vi "Main.vi"() -> ()   [LabVIEW 2021]
doc: "Use this template to build a simple state machine design pattern. Each state executes code and determines which state to transition to."
uses:
  controls/UI Data.ctl
  Serial - Settings.ctl
  controls/Sensor parameters.ctl
  controls/State.ctl
  dd997a8f-e2f9-4ff0-8e35-442db1fc508d.vi
  22f98573-57d9-4471-b3a5-586873744a38.vi
  <vilib>/Instr/_visa.llb/VISA Configure Serial Port (Instr).vi
  <vilib>/Utility/file.llb/Write Delimited Spreadsheet (string).vi
panel:
  in  "AUTOMATICKE NASTAVENI \nPARAMETRU":enum16{"OFF", "Presnost", "Rychlost"}(ring)
  in  "Tab Control":T1(tab)
  in  "Ukladani":u16(ring) items=[".csv", ".tdms"]
  in  "Celkovy pocet mereni":u32=20 step=10
  in  "Pocet mereni na prumer":u32=5 min=1 max=20
  in  "Pocet mereni za sekundu":dbl=4.0 min=1.0 max=5.0
  in  "Save measurement to:":path=path "TEST3"
  in  "VISA resource name 34450A":refnum<visa-resource-name>="key"
  in  "delay before read 34450A":u32=500
  in  "Rozsah 34450A":T2(ring)=enum."10 V"
  in  "Rozliseni 34450A":enum16{"4_1/2 fast", "4_1/2 slow", "5_1/2 fast"}(ring)
  in  "VISA resource name 34401A":refnum<visa-resource-name>="COM7"
  in  "delay before read 34401A":u32=500
  in  "Rozliseni 34401A":T3(ring)
  in  "Rozsah 34401A":enum16{"10 mA", "100 mA", "1 A", "3 A"}(ring)
  in  "Serial Settings 34401A":T4={"baud rate"=9600, "data bits"=8, "parity"=enum."None", "stop bits"=10, "flow control"=0} {"flow control" items=["None"=0, "XON/XOFF"=1, "RTS/CTS"=2, "DTR/DSR"=4]; "stop bits" items=["1.0"=10, "1.5"=15, "2.0"=20]; "data bits" min=5 max=8 step=1; "baud rate" items=["75"=75, "110"=110, "134"=134, "150"=150, "300"=300, "600"=600, "1200"=1200, "1800"=1800, "2400"=2400, "4800"=4800, "7200"=7200, "9600"=9600, "14400"=14400, "19200"=19200, "28800"=28800, "38400"=38400, "56000"=56000, "57600"=57600, "115200"=115200, "128000"=128000, "230400"=230400]}
  out "Odhad konce mereni":timestamp
  out "Start mereni":timestamp
  in  "Stop mereni":bool
  out "Probiha mereni":u8(slide) scale=0.0..1.0
  in  "Sensor parameters":T5
  in  "Start mereni":bool
  out "Prumerna teplota":waveform(dbl)(graph)={"t0"=timestamp(3860297685.555485 s since 1904-01-01), "dt"=1.2529971599578857, "Y"=[-inf, -inf, -inf, -inf, nan]}
  out "Table":string[][](table)=[["Casy prumeru", "4/29/2026 10:54:45 AM", "4/29/2026 10:54:46 AM", "4/29/2026 10:54:48 AM", "4/29/2026 10:54:49 AM", "2/28/1965 5:27:24 PM"], ["Prumery napeti [V]", "-0.000417", "-0.000469", "-0.000557", "-0.000539", "NaN"], ["Prumery proudu [A]", "-0.000000", "0.000000", "-0.000000", "-0.000001", "NaN"], ["Prumery odporu [Ohm]", "-10579.900593", "-10579.900593", "-10579.900593", "-10579.900593", "NaN"], ["Prumery teploty [°C]", "-Inf", "-Inf", "-Inf", "-Inf", "NaN"], ["Nejistoty teplot [°C]", "NaN", "NaN", "NaN", "NaN", "NaN"]]
  in  "stop":bool
  in  "Data":T6={"VISA resource name 34401A"="COM1", "Serial Settings 34401A"={"baud rate"=9600, "data bits"=8, "parity"=enum."None", "stop bits"=10, "flow control"=0}, "VISA resource name 34450"="COM1", "VISA OUT 34401A"="", "VISA OUT 34450"="", "Delay before read 34401A"=0, "Delay before read 34450"=0, "Pocet mereni za sekundu"=1.0, "Celkovy pocet mereni"=1, "Pocet mereni na prumer"=1, "Rozliseni 34401A"=enum."4_1/2 fast", "Rozliseni 34450"=enum."5_1/2 fast", "AUTOMATICKE NASTAVENI \nPARAMETRU"=enum."OFF", "Namerene napeti"=[], "Namerene proudy"=[], "Prumery napeti"=[], "Prumery proudu"=[], "Namerene odpory"=[], "Namerene teploty"=[], "Prumery odporu"=[], "Prumery teplot"=[], "Rozsah 34401A"=enum."10 mA", "Rozsah 34450"=enum."100 mV", "Sensor parameters"={"Sensor type"="", "Sensor constant"=0.0}, "Casy mereni"=[], "Casy prumerovani"=[], "Nejistoty teplot"=[]} {"Pocet mereni na prumer" min=1; "Celkovy pocet mereni" min=1 max=5; "Serial Settings 34401A"."flow control" items=["None"=0, "XON/XOFF"=1, "RTS/CTS"=2, "DTR/DSR"=4]; "Serial Settings 34401A"."stop bits" items=["1.0"=10, "1.5"=15, "2.0"=20]; "Serial Settings 34401A"."data bits" min=5 max=8 step=1; "Serial Settings 34401A"."baud rate" items=["75"=75, "110"=110, "134"=134, "150"=150, "300"=300, "600"=600, "1200"=1200, "1800"=1800, "2400"=2400, "4800"=4800, "7200"=7200, "9600"=9600, "14400"=14400, "19200"=19200, "28800"=28800, "38400"=38400, "56000"=56000, "57600"=57600, "115200"=115200, "128000"=128000, "230400"=230400]}
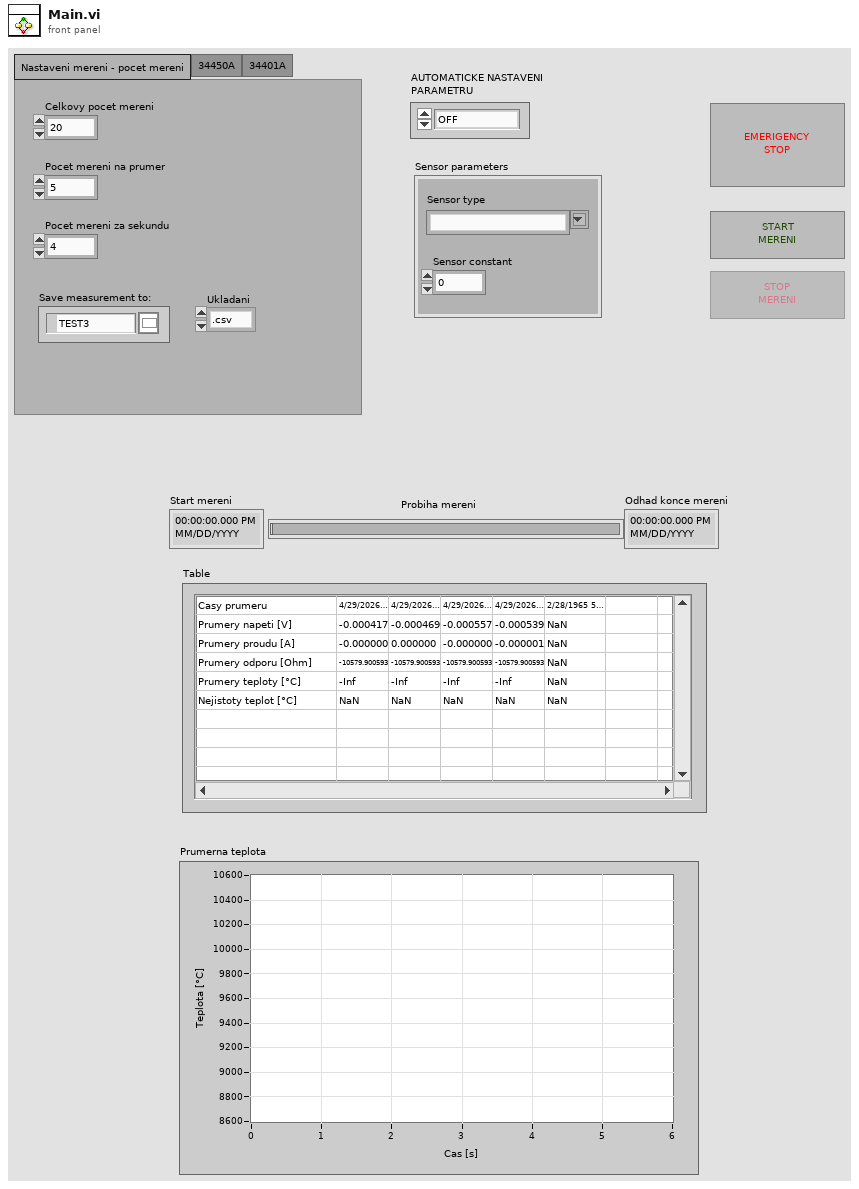
[diagram p1: front panel]
types:
  T1 = enum32{"Nastaveni mereni - pocet mereni", "34450A", "34401A"}
  T2 = enum16{"100 mV", "1 V", "10 V", "100 V", "1000 V"}
  T3 = enum16{"4_1/2 fast", "4_1/2 slow", "5_1/2 fast", "5_1/2 slow", "6_1/2 fast", "6_1/2 slow"}
  T4 = typedef "Serial - Settings.ctl" = cluster{"baud rate":u32, "data bits":u16, "parity":enum16{"None", "Odd", "Even", "Mark", "Space"}, "stop bits":u16, "flow control":u16}
  T5 = typedef "Sensor parameters.ctl" = cluster{"Sensor type":string, "Sensor constant":dbl}
  T6 = typedef "UI Data.ctl" = cluster{"VISA resource name 34401A":refnum<visa-resource-name>, "Serial Settings 34401A":T4, "VISA resource name 34450":refnum<visa-resource-name>, "VISA OUT 34401A":refnum<visa-resource-name>, "VISA OUT 34450":refnum<visa-resource-name>, "Delay before read 34401A":u32, "Delay before read 34450":u32, "Pocet mereni za sekundu":dbl, "Celkovy pocet mereni":u32, "Pocet mereni na prumer":u32, "Rozliseni 34401A":enum16{"4_1/2 fast", "4_1/2 slow", "5_1/2 fast", "5_1/2 slow", "6_1/2 fast", "6_1/2 slow"}, "Rozliseni 34450":enum16{"4_1/2 fast", "4_1/2 slow", "5_1/2 fast"}, "AUTOMATICKE NASTAVENI \nPARAMETRU":enum16{"OFF", "Presnost", "Rychlost"}, "Namerene napeti":dbl[], "Namerene proudy":dbl[], "Prumery napeti":dbl[], "Prumery proudu":dbl[], "Namerene odpory":dbl[], "Namerene teploty":dbl[], "Prumery odporu":dbl[], "Prumery teplot":dbl[], "Rozsah 34401A":enum16{"10 mA", "100 mA", "1 A", "3 A"}, "Rozsah 34450":enum16{"100 mV", "1 V", "10 V", "100 V", "1000 V"}, "Sensor parameters":T5, "Casy mereni":timestamp[], "Casy prumerovani":timestamp[], "Nejistoty teplot":dbl[]}
  T7 = typedef "State.ctl" = enum16{"Boot", "Set_params", "Initialization", "Measure", "Math", "Display", "Meas_done?", "Meas_end", "High_level_math", "Save_param", "Save_measure"}
  T8 = enum8{"Enabled", "Disabled", "Disabled and Grayed Out"}
  T9 = enum16{"OFF", "Pt 100 presnost", "Pt 100 rychlost", "Pt 1000 presnost", "Pt 1000 rychlost"}
  T10 = enum16{"open", "open or create", "create or replace", "create", "open (read-only)"}
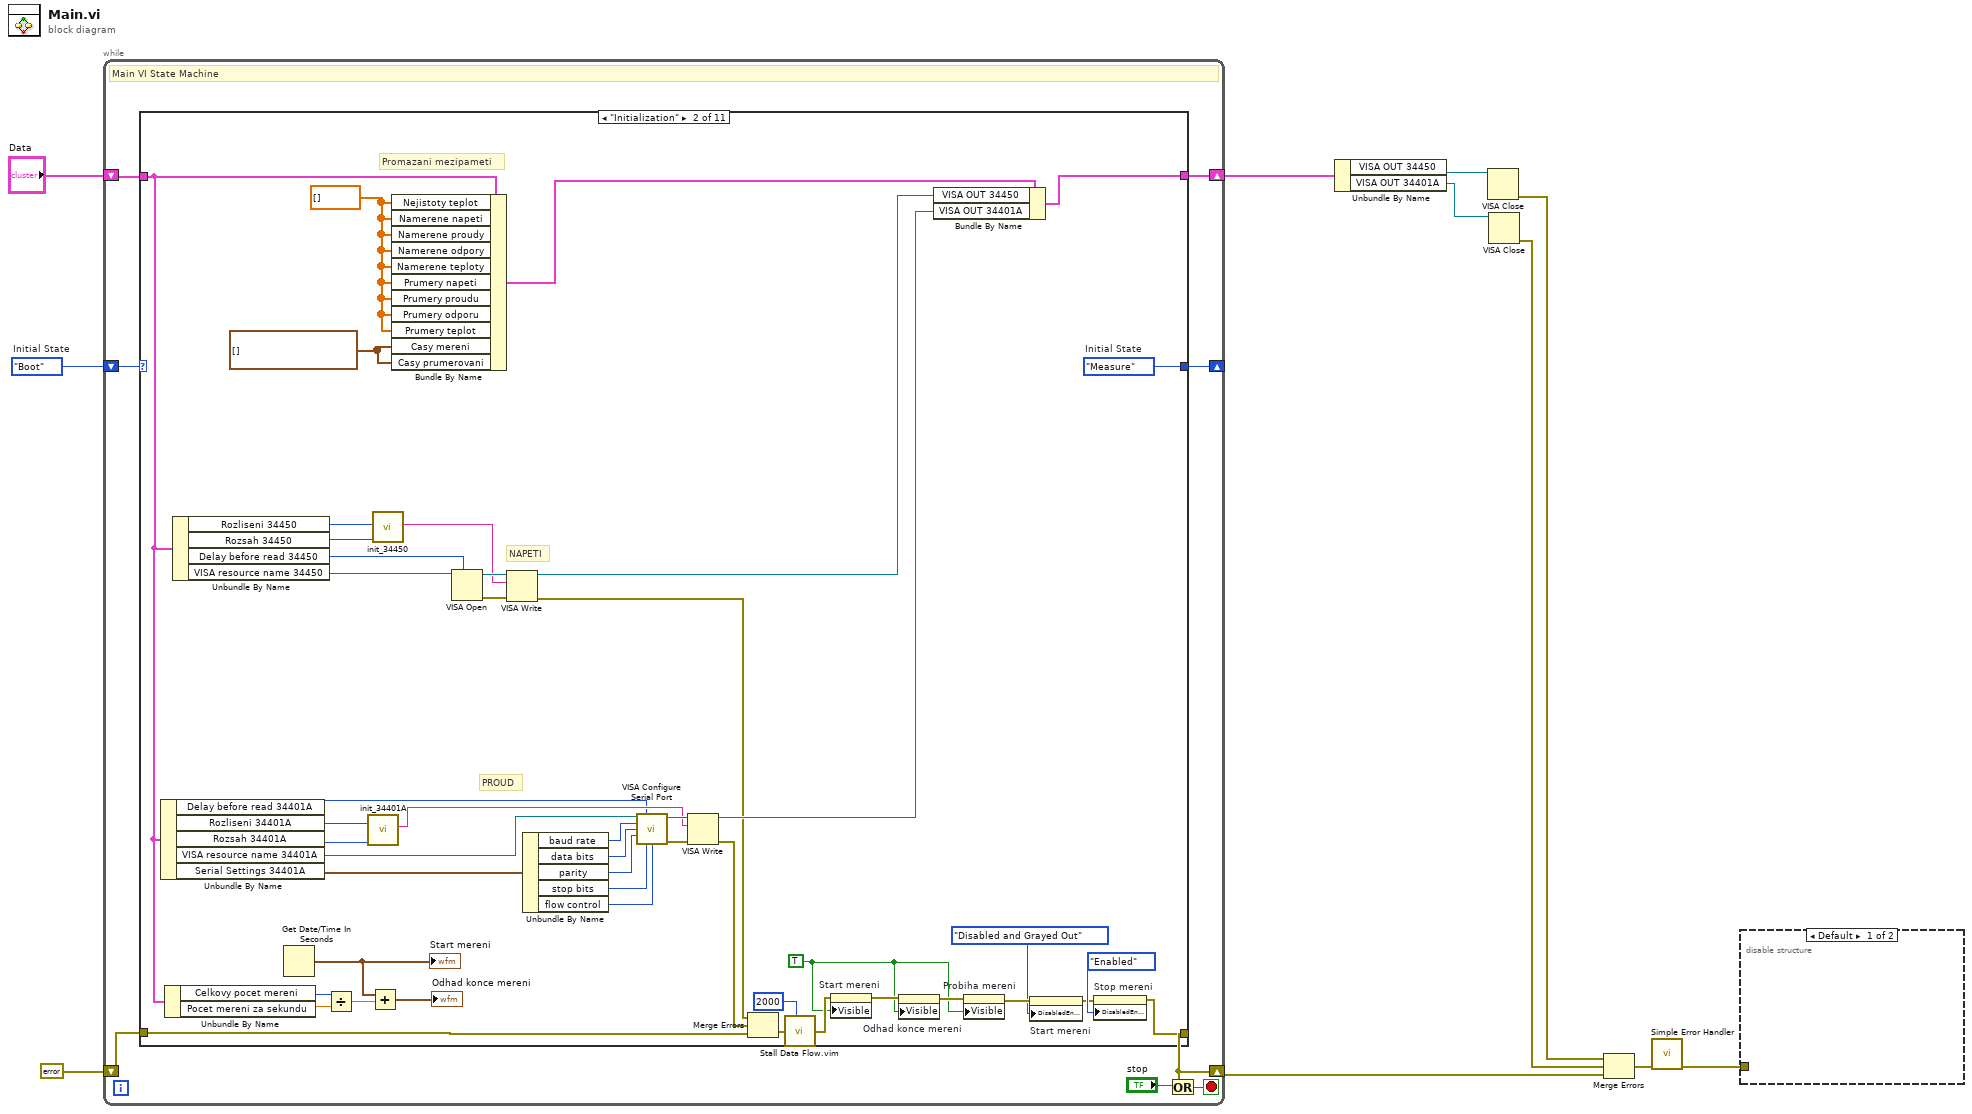
[diagram p0: block diagram]
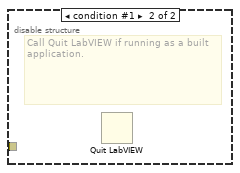
[diagram p2: hidden frame]
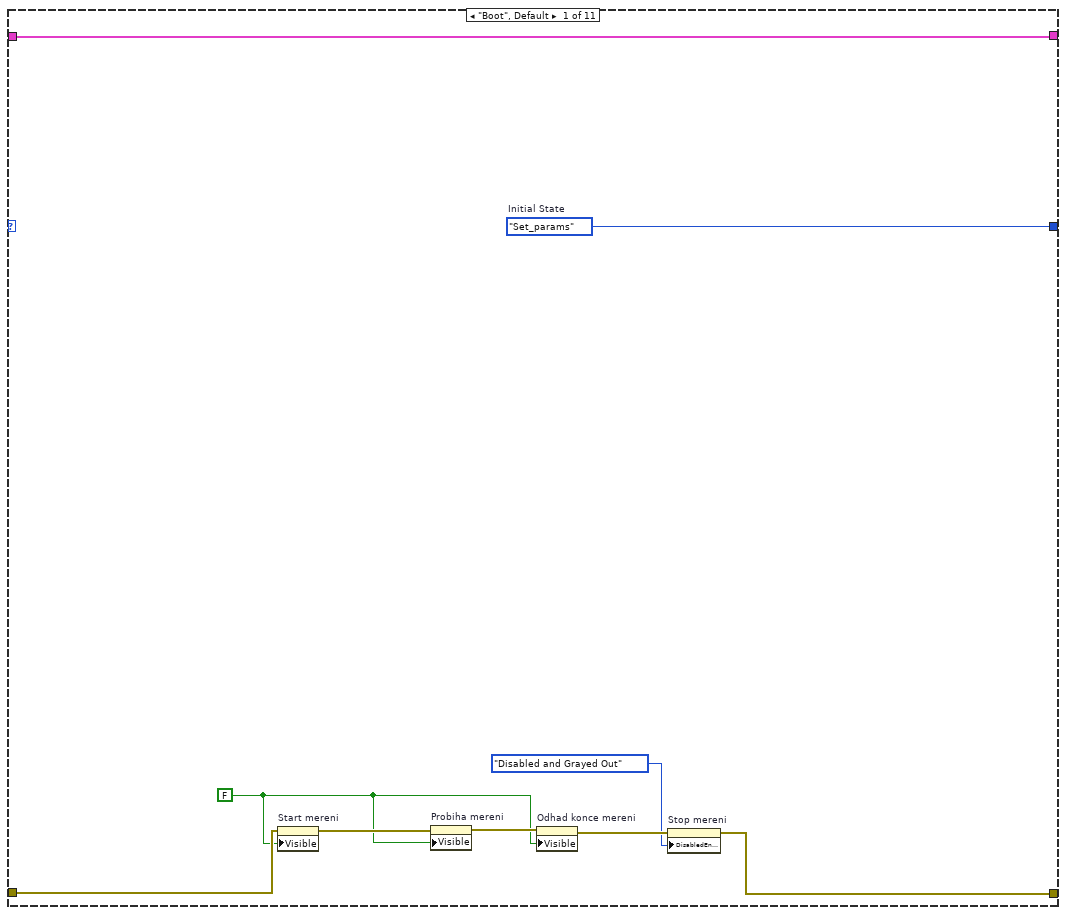
[diagram p3: hidden frame]
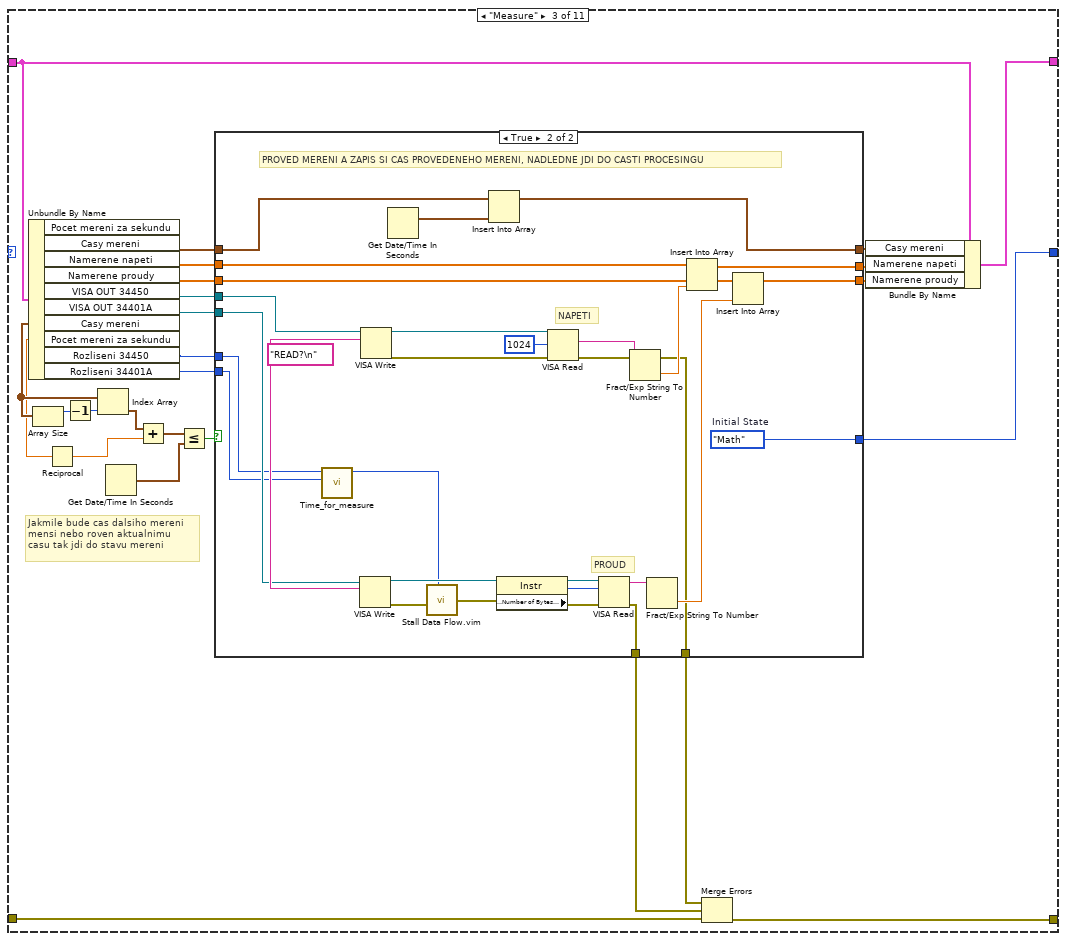
[diagram p4: hidden frame]
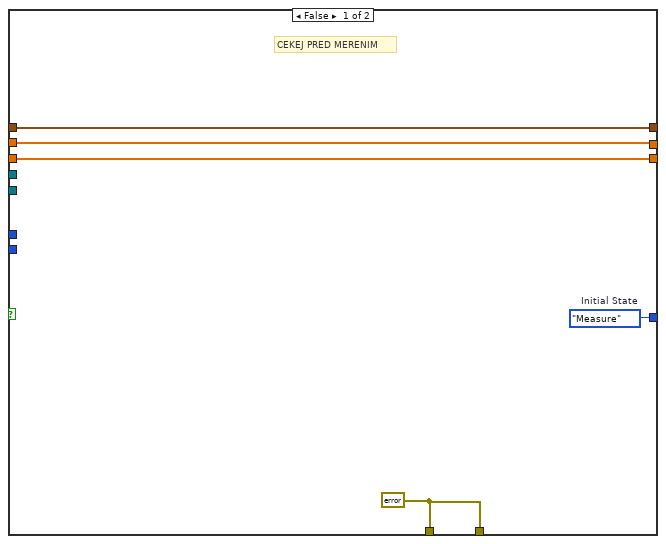
[diagram p5: hidden frame]
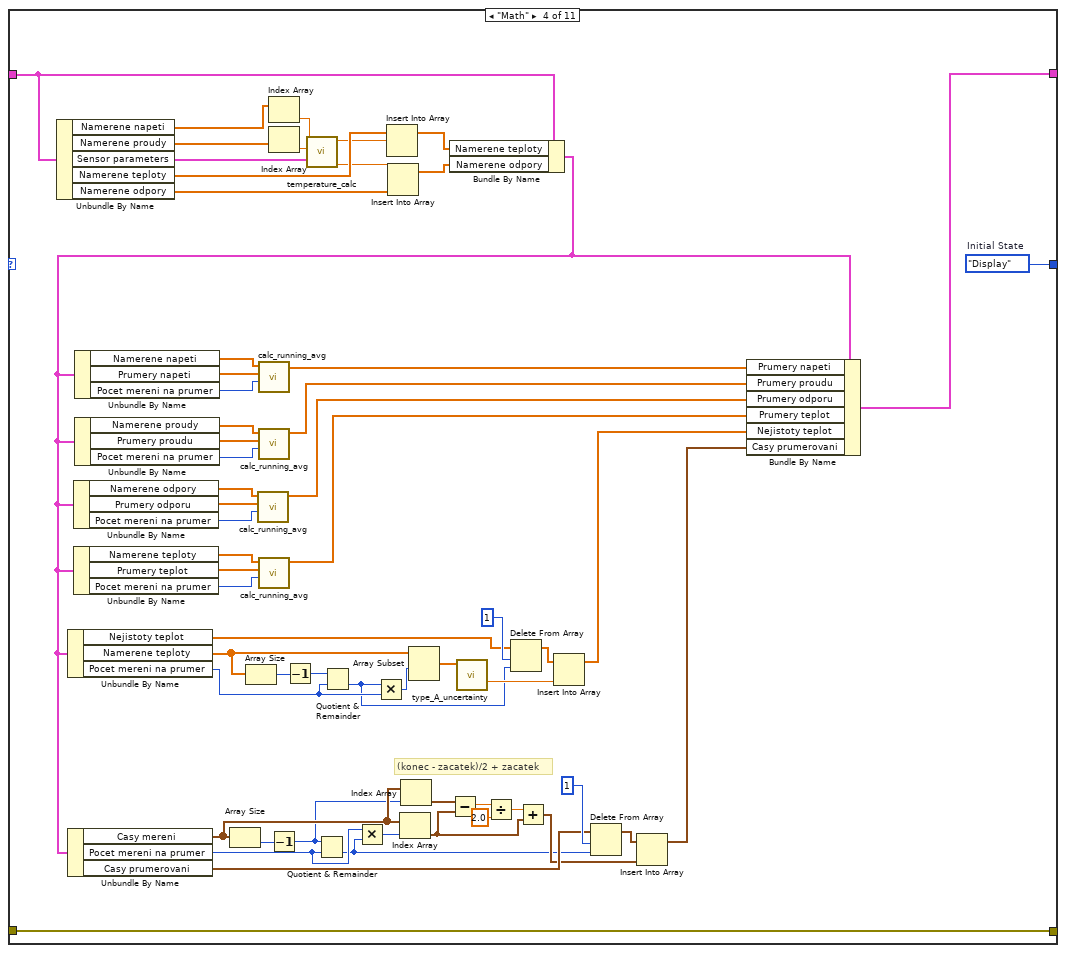
[diagram p6: hidden frame]
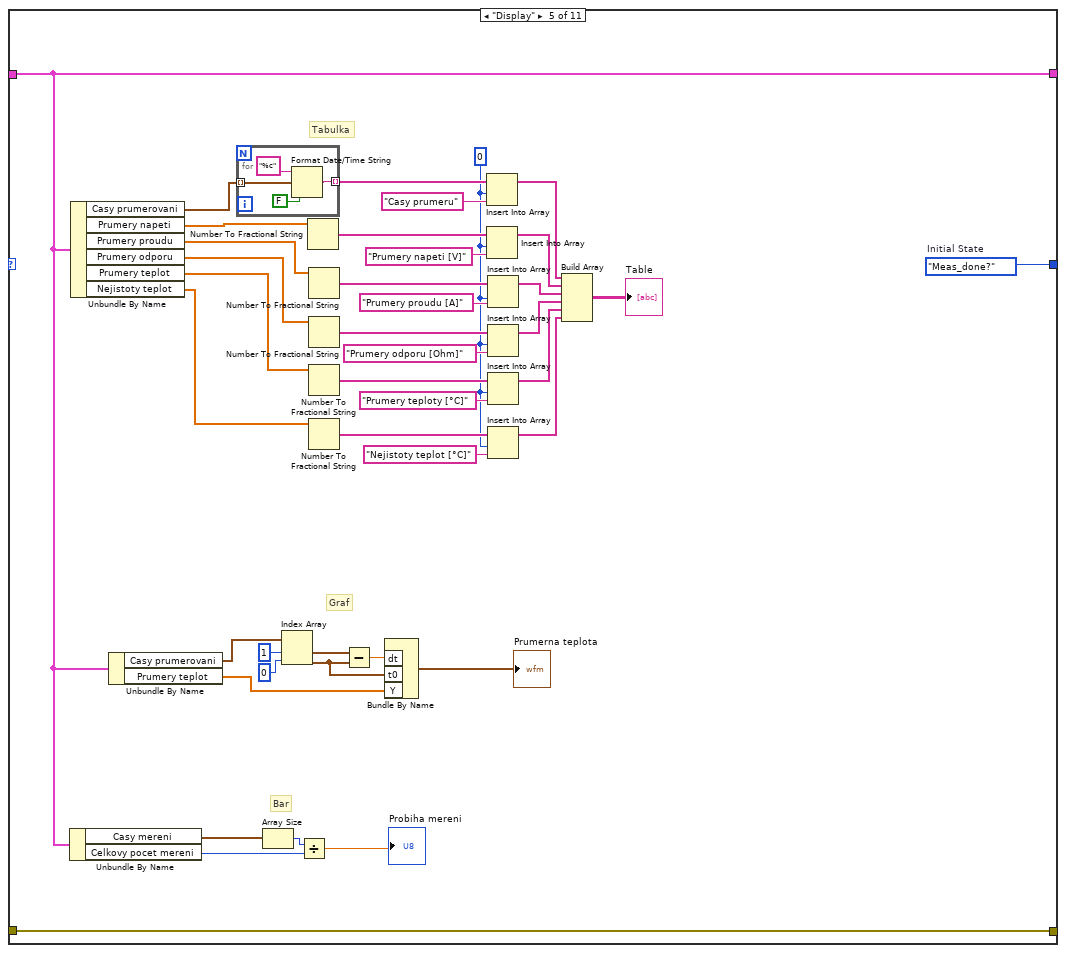
[diagram p7: hidden frame]
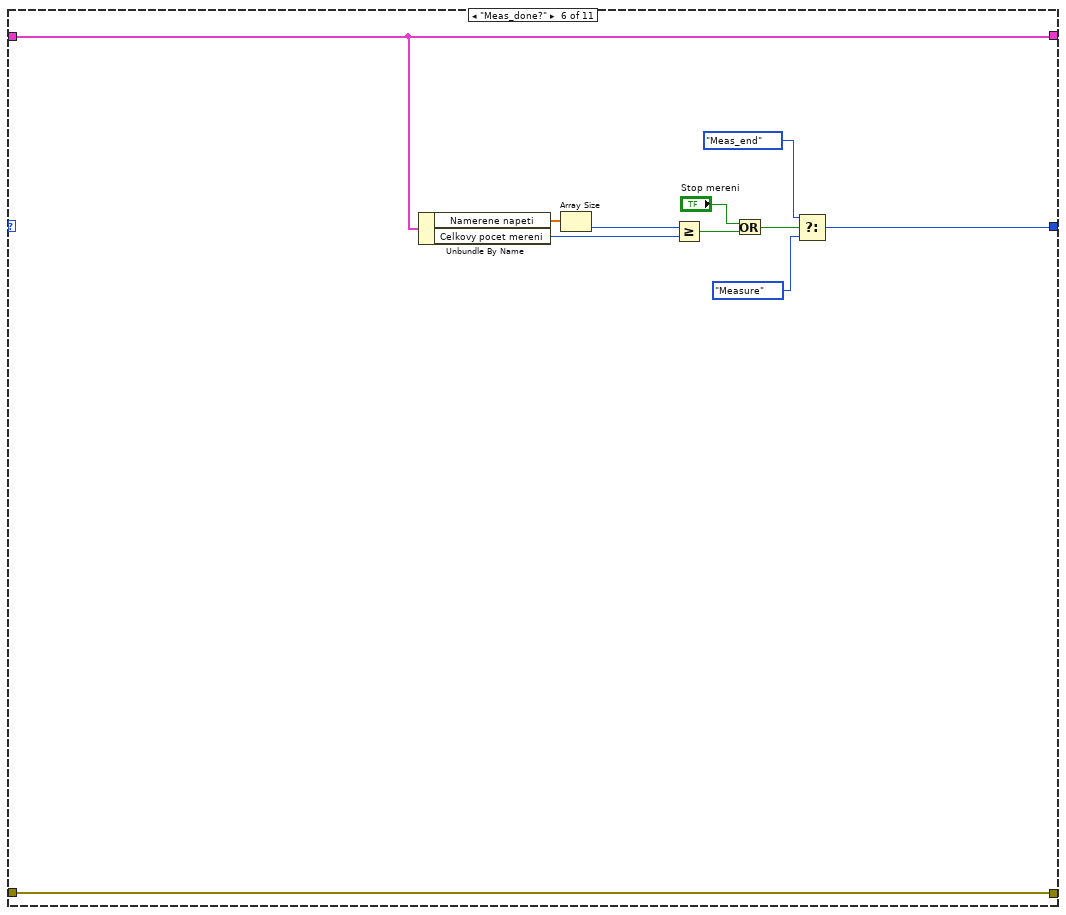
[diagram p8: hidden frame]
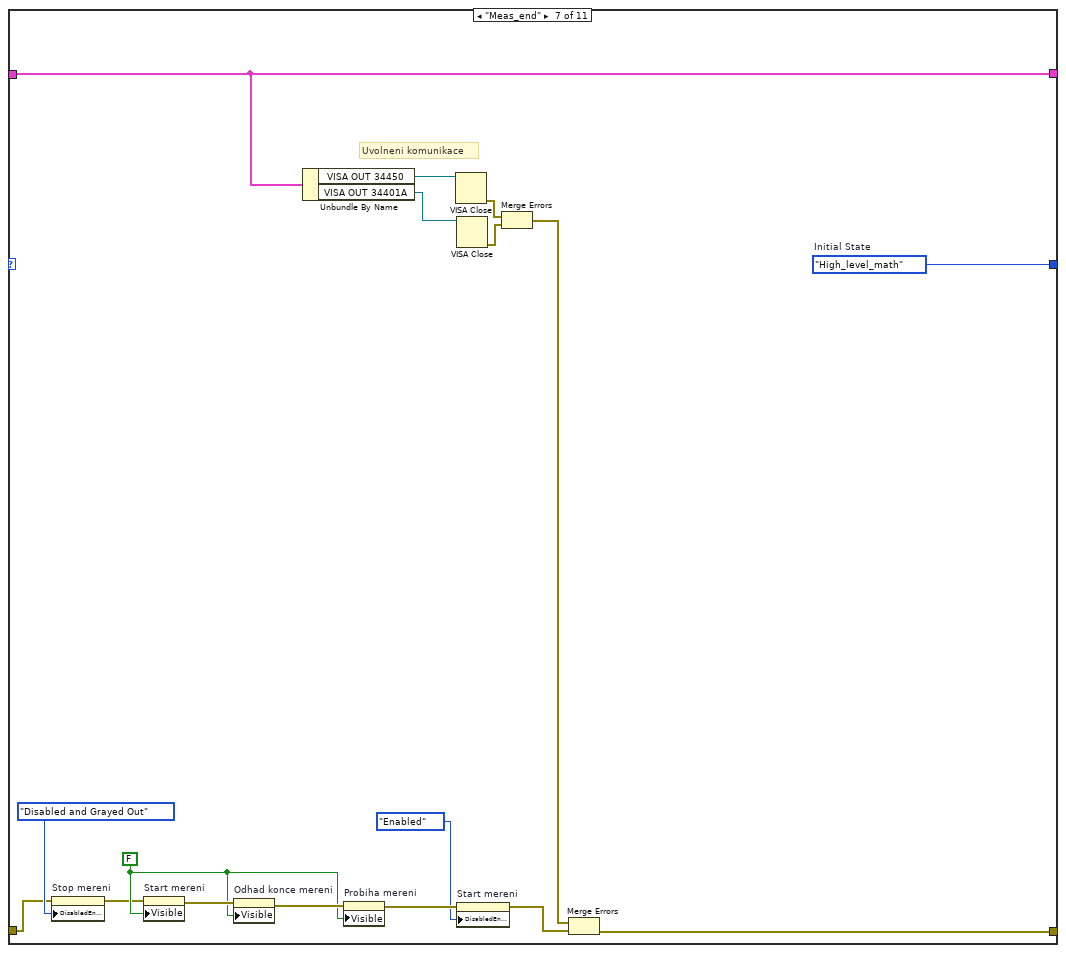
[diagram p9: hidden frame]
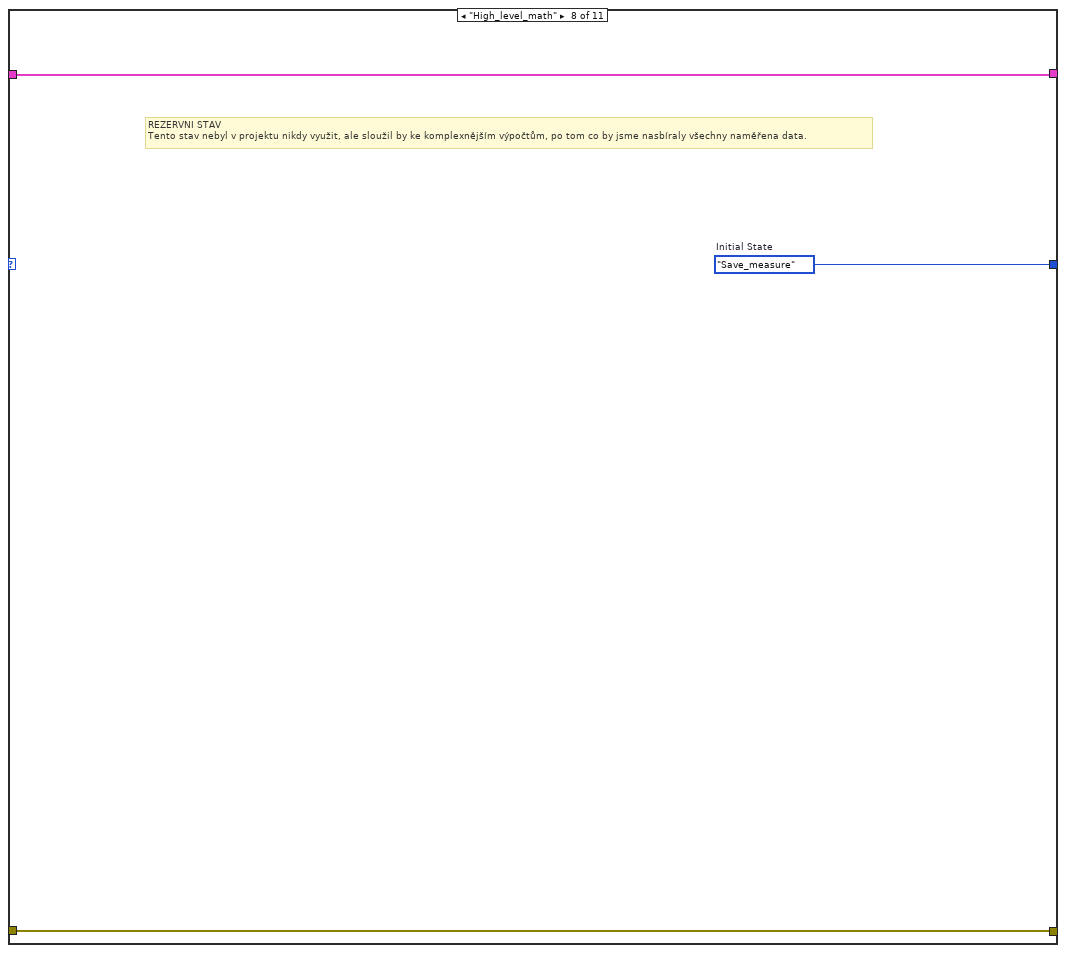
[diagram p10: hidden frame]
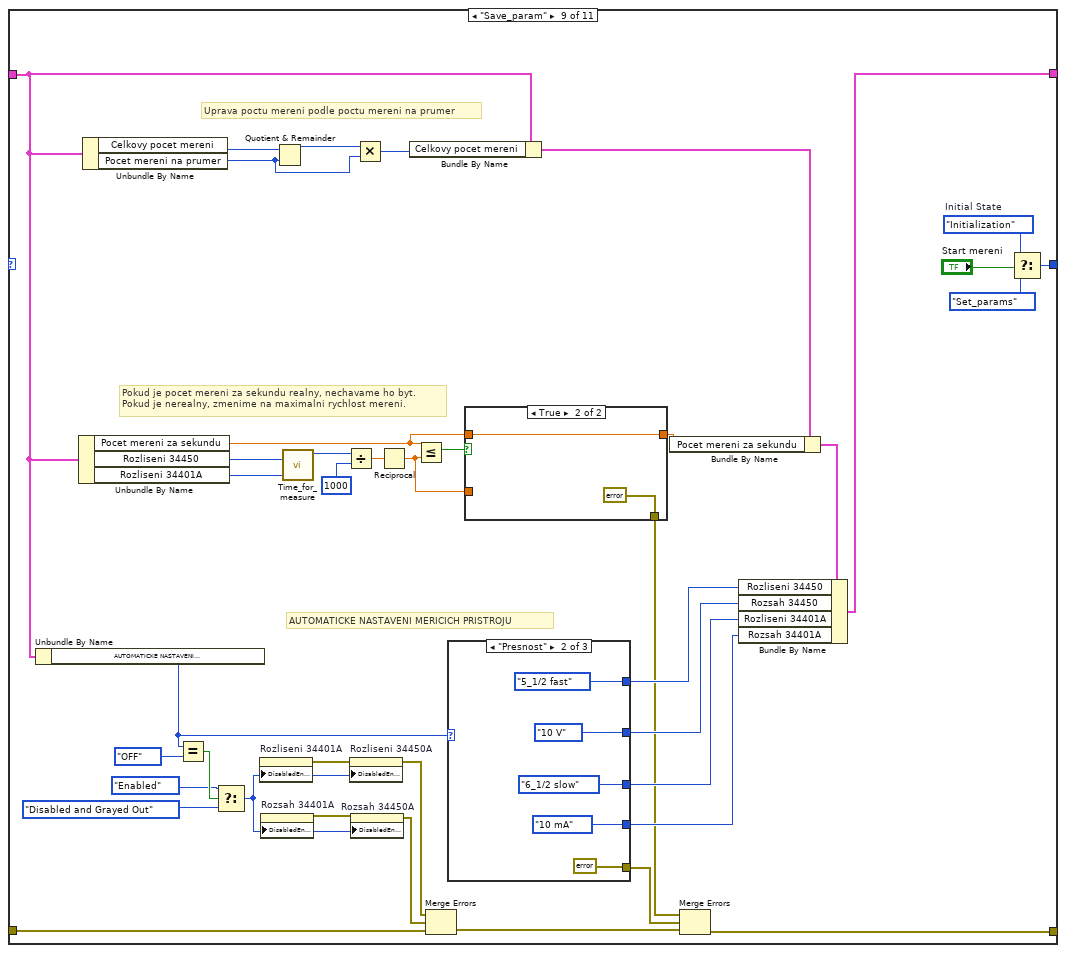
[diagram p11: hidden frame]
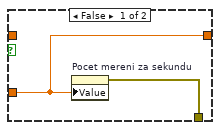
[diagram p12: hidden frame]
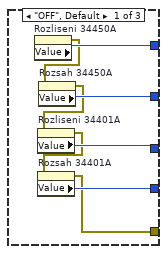
[diagram p13: hidden frame]
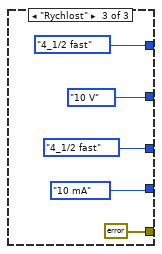
[diagram p14: hidden frame]
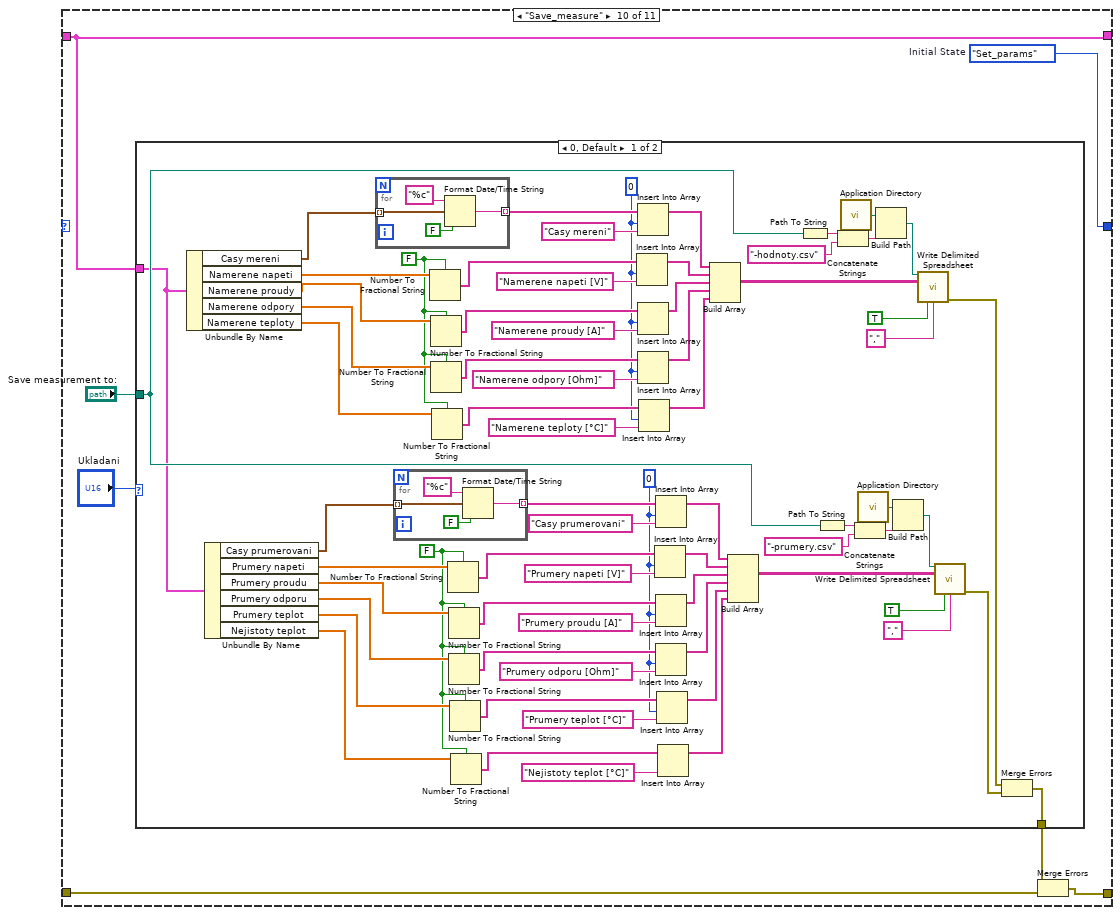
[diagram p15: hidden frame]
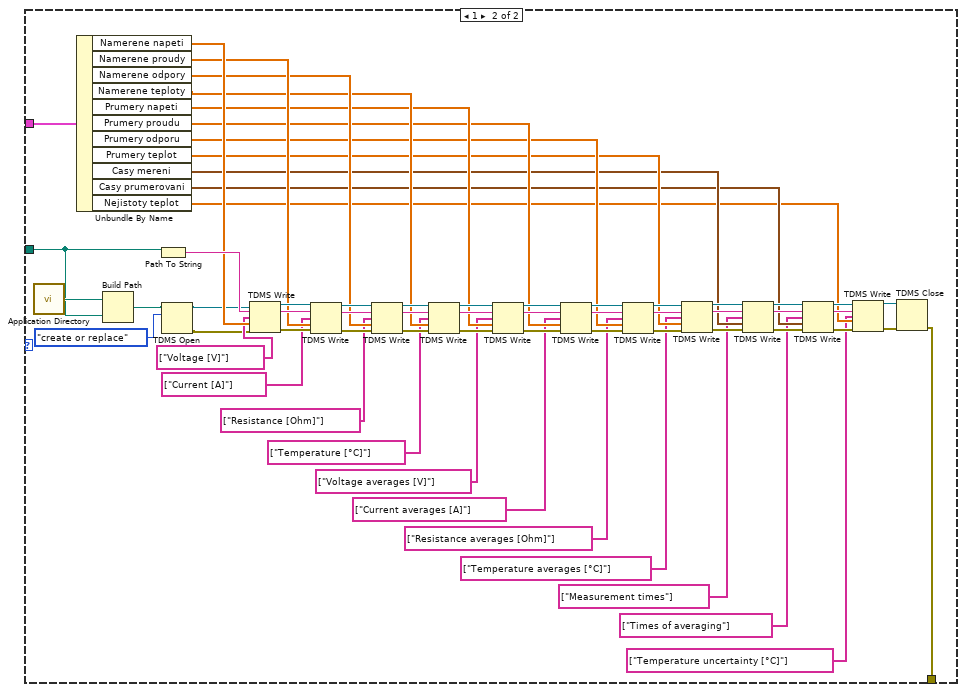
[diagram p16: hidden frame]
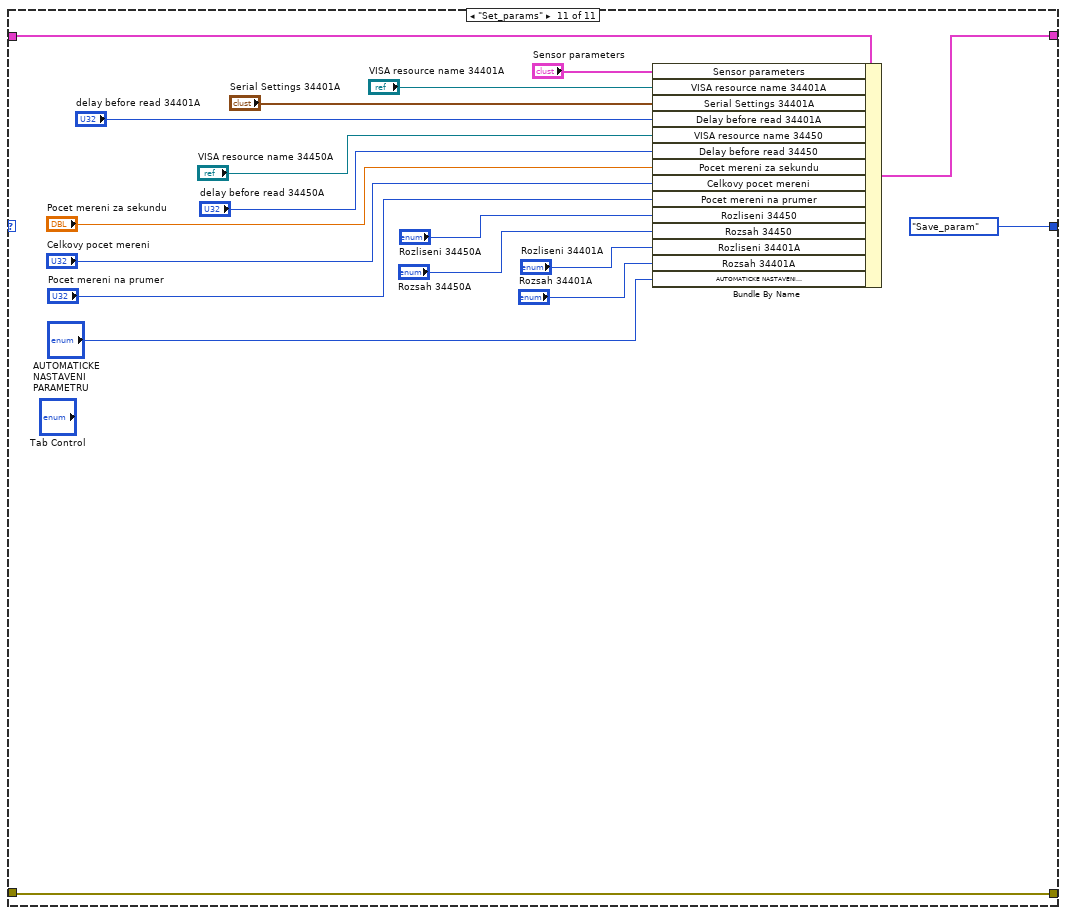
[diagram p17: hidden frame]
diagram:
  w11 = State."Boot"  # Initial State
  n1 = while {
    shift-right: [w14] -> _
    shift-left: w11 -> [w18]
    shift-right: [w13] -> w7
    shift-left: "Data" -> [w17]
    shift-right: [w15] -> w4
    shift-left: errorcluster {"status"=FALSE, "code"=0, "source"=""} ("error constant") -> [w16]
    stop <- w19 stop-if-true
    # "Main VI State Machine"
    n2 = case shown="\"Initialization\"" w18 {
      tunnel: w17 -> [w28 w44 w99 w184 w200 w250 w265 w269 w289 w340 w498]
      tunnel: w16 -> [w26 w38 w96 w195 w236 w251 w258 w271 w291 w339 w483]
      tunnel: [w21 w33 w95 w195 w236 w251 w264 w271 w303 w338 w483] -> w15
      tunnel: [w27 w75 w101 w194 w206 w246 w268 w270 w296 w336 State."Save_param" ("Initial State")] -> w14
      tunnel: [w28 w65 w98 w165 w200 w250 w265 w269 w278 w340 w497] -> w13
      frame "Boot", Default {
        w23 = FALSE ("Visible")
        w27 = State."Set_params"  # Initial State
        n3 = property on="Start mereni" class="AbsTime (strict)"(error in=w26, "Visible"=w23) -> (error out=w25:errorcluster)  [unwired: 1 in, 1 out]
        n4 = property on="Probiha mereni" class="Slide (strict)"(error in=w25, "Visible"=w23) -> (error out=w24:errorcluster)  [unwired: 1 in, 1 out]
        n5 = property on="Odhad konce mereni" class="AbsTime (strict)"(error in=w24, "Visible"=w23) -> (error out=w22:errorcluster)  [unwired: 1 in, 1 out]
        n6 = property on="Stop mereni" class="Bool"(error in=w22, "DisabledEnum"=T8."Disabled and Grayed Out" ("Disabled")) -> (error out=w21:errorcluster)  [unwired: 1 in, 1 out]
      }
      frame "Initialization" {
        w34 = TRUE ("Visible")
        w45 = dbl[] [] ("Namerene napeti")
        w47 = timestamp[] [] ("Casy mereni")
        w75 = State."Measure"  # Initial State
        # "Promazani mezipameti"
        # "PROUD"
        # "NAPETI"
        n7 = Unbundle By Name(w44) -> ("Delay before read 34401A"=w50:u32, "Rozliseni 34401A"=w56:T3, "Rozsah 34401A"=w53:enum16{"10 mA", "100 mA", "1 A", "3 A"}, "VISA resource name 34401A"=w67:refnum<visa-resource-name>, "Serial Settings 34401A"=w66:T4)
        n8 = Unbundle By Name(w44) -> ("Celkovy pocet mereni"=w43:u32, "Pocet mereni za sekundu"=w42:dbl)
        n9 = Unbundle By Name(w44) -> ("Rozliseni 34450"=w58:enum16{"4_1/2 fast", "4_1/2 slow", "5_1/2 fast"}, "Rozsah 34450"=w54:T2, "Delay before read 34450"=w51:u32, "VISA resource name 34450"=w52:refnum<visa-resource-name>)
        n10 = Get Date/Time In Seconds() -> (seconds since 1Jan1904=w41:timestamp)
        "Start mereni" <- w41
        n11 = Divide(x=w43, y=w42) -> (x/y=w40:dbl)
        n12 = call "init_34401A.vi"("Rozsah 34401A"=w53, "Rozliseni 34401A"=w56) -> ("Command String"=w55:string)  [unwired: 9 in]
        n13 = Add(x=w41, y=w40) -> (x+y=→"Odhad konce mereni":timestamp)
        n14 = call "init_34450.vi"("Rozsah 3450A"=w54, "Rozliseni 34450"=w58) -> ("Command String"=w57:string)  [unwired: 9 in]
        n15 = Bundle By Name(cluster=w44, "Nejistoty teplot"=w45, "Namerene napeti"=w45, "Namerene proudy"=w45, "Namerene odpory"=w45, "Namerene teploty"=w45, "Prumery napeti"=w45, "Prumery proudu"=w45, "Prumery odporu"=w45, "Prumery teplot"=w45, "Casy mereni"=w47, "Casy prumerovani"=w47) -> (w46:T6)
        n16 = VISA Open(timeout (0)=w51, VISA resource name=w52) -> (VISA resource name=w63:refnum<visa-resource-name>, error out=w61:errorcluster)  [unwired: 3 in]
        n17 = VISA Write(VISA resource name=w63, write buffer=w57, error in (no error)=w61) -> (VISA resource name out=w62:refnum<visa-resource-name>, error out=w59:errorcluster)  [unwired: 1 out]
        n18 = Unbundle By Name(w66) -> ("baud rate"=w72:u32, "data bits"=w71:u16, "parity"=w70:enum16{"None", "Odd", "Even", "Mark", "Space"}, "stop bits"=w69:u16, "flow control"=w68:u16)
        n19 = call-poly "VISA Configure Serial Port"("VISA resource name"=w67, "timeout (10sec)"=w50, "baud rate (9600)"=w72, "data bits (8)"=w71, "parity (0:none)"=w70, "stop bits (10: 1 bit)"=w69, "flow control (0:none)"=w68) -> ("VISA resource name out"=w73:refnum<visa-resource-name>, "error out"=w74:errorcluster)  [unwired: 2 in, 5 out]
        n20 = VISA Write(VISA resource name=w73, write buffer=w55, error in (no error)=w74) -> (VISA resource name out=w64:refnum<visa-resource-name>, error out=w60:errorcluster)  [unwired: 1 out]
        n21 = Merge Errors(w59, w60, w38) -> (w49:errorcluster)
        n22 = call "Stall Data Flow.vim"("value in"=w49, "milliseconds to wait"=u32 2000) -> ("value out"=w35:errorcluster)  [unwired: 1 out]
        n23 = property on="Start mereni" class="AbsTime (strict)"(error in=w35, "Visible"=w34) -> (error out=w37:errorcluster)  [unwired: 1 in, 1 out]
        n24 = property on="Odhad konce mereni" class="AbsTime (strict)"(error in=w37, "Visible"=w34) -> (error out=w36:errorcluster)  [unwired: 1 in, 1 out]
        n25 = Bundle By Name(cluster=w46, "VISA OUT 34450"=w62, "VISA OUT 34401A"=w64) -> (w65:T6)
        n26 = property on="Probiha mereni" class="Slide (strict)"(error in=w36, "Visible"=w34) -> (error out=w30:errorcluster)  [unwired: 1 in, 1 out]
        n27 = property on="Start mereni" class="Bool"(error in=w30, "DisabledEnum"=T8."Disabled and Grayed Out" ("Disabled")) -> (error out=w31:errorcluster)  [unwired: 1 in, 1 out]
        n28 = property on="Stop mereni" class="Bool"(error in=w31, "DisabledEnum"=T8."Enabled" ("Disabled")) -> (error out=w33:errorcluster)  [unwired: 1 in, 1 out]
      }
      frame "Measure" {
        # "Jakmile bude cas dalsiho mereni\nmensi nebo roven aktualnimu\ncasu tak jdi do stavu mereni"
        n29 = Unbundle By Name(w99) -> ("Casy mereni"=w87:timestamp[], "Namerene napeti"=w93:dbl[], "Namerene proudy"=w92:dbl[], "VISA OUT 34450"=w100:refnum<visa-resource-name>, "VISA OUT 34401A"=w97:refnum<visa-resource-name>, "Casy mereni"=w85:timestamp[], "Pocet mereni za sekundu"=w84:dbl, "Rozliseni 34450"=w76:enum16{"4_1/2 fast", "4_1/2 slow", "5_1/2 fast"}, "Rozliseni 34401A"=w77:T3)  [unwired: 1 out]
        n30 = Array Size(array=w85) -> (size(s)=w86:i32)
        n31 = Reciprocal(x=w84) -> (1/x=w82:dbl)
        n32 = Decrement(x=w86) -> (x-1=w78:i32)
        n33 = Index Array(array=w85, index=w78) -> (element=w83:timestamp)
        n34 = Get Date/Time In Seconds() -> (seconds since 1Jan1904=w80:timestamp)
        n35 = Add(x=w83, y=w82) -> (x+y=w81:timestamp)
        n36 = Less Or Equal?(x=w81, y=w80) -> (x <= y?=w79:bool)
        n37 = case shown="True" w79 {
          tunnel: [w103 w135] -> w101
          tunnel: w100 -> [_ w131]
          tunnel: w97 -> [_ w110]
          tunnel: [w102 w124] -> w94
          tunnel: w93 -> [w105 w123]
          tunnel: w92 -> [w104 w122]
          tunnel: [w104 w119] -> w91
          tunnel: [w105 w118] -> w90
          tunnel: [w102 w117] -> w89
          tunnel: [w106 w114] -> w88
          tunnel: w87 -> [w106 w116]
          tunnel: w77 -> [_ w109]
          tunnel: w76 -> [_ w108]
          frame False {
            w102 = errorcluster {"status"=FALSE, "code"=0, "source"=""} ("error constant")
            w103 = State."Measure"  # Initial State
            # "CEKEJ PRED MERENIM"
          }
          frame True {
            w130 = "READ?\n" ("Command")
            w135 = State."Math"  # Initial State
            # "PROVED MERENI A ZAPIS SI CAS PROVEDENEHO MERENI, NADLEDNE JDI DO CASTI PROCESINGU"
            # "PROUD"
            # "NAPETI"
            n38 = call "Time_for_measure.vi"("Rozliseni 34401A"=w109, "Rozliseni 34450"=w108) -> ("Time for measure"=w107:u32)  [unwired: 9 in]
            n39 = VISA Write(VISA resource name=w110, write buffer=w130) -> (VISA resource name out=w111:refnum<visa-resource-name>, error out=w113:errorcluster)  [unwired: 1 in, 1 out]
            n40 = VISA Write(VISA resource name=w131, write buffer=w130) -> (VISA resource name out=w127:refnum<visa-resource-name>, error out=w125:errorcluster)  [unwired: 1 in, 1 out]
            n41 = Get Date/Time In Seconds() -> (seconds since 1Jan1904=w115:timestamp)
            n42 = call "Stall Data Flow.vim"("value in"=w113, "milliseconds to wait"=w107) -> ("value out"=w112:errorcluster)  [unwired: 1 out]
            n43 = Insert Into Array(array=w116, new element=w115) -> (w114:timestamp[])  [unwired: 1 in]
            n44 = property class="Instr"(reference=w111, error in=w112) -> (reference out=w134:refnum<visa-resource-name>, error out=w133:errorcluster, "Serial Settings:Number of Bytes at Serial Port"=w132:u32)
            n45 = VISA Read(VISA resource name=w127, byte count=u32 1024, error in (no error)=w125) -> (read buffer=w129:string, error out=w117:errorcluster)  [unwired: 2 out]
            n46 = VISA Read(VISA resource name=w134, byte count=w132, error in (no error)=w133) -> (read buffer=w128:string, error out=w124:errorcluster)  [unwired: 2 out]
            n47 = Fract/Exp String To Number(string=w129) -> (number=w121:dbl)  [unwired: 3 in, 1 out]
            n48 = Fract/Exp String To Number(string=w128) -> (number=w120:dbl)  [unwired: 3 in, 1 out]
            n49 = Insert Into Array(array=w123, new element=w121) -> (w118:dbl[])  [unwired: 1 in]
            n50 = Insert Into Array(array=w122, new element=w120) -> (w119:dbl[])  [unwired: 1 in]
          }
        }
        n51 = Merge Errors(w89, w94, w96) -> (w95:errorcluster)
        n52 = Bundle By Name(cluster=w99, "Casy mereni"=w88, "Namerene napeti"=w90, "Namerene proudy"=w91) -> (w98:T6)
      }
      frame "Math" {
        w194 = State."Display"  # Initial State
        # "(konec - zacatek)/2 + zacatek"
        n53 = Unbundle By Name(w184) -> ("Namerene napeti"=w193:dbl[], "Namerene proudy"=w192:dbl[], "Sensor parameters"=w189:T5, "Namerene teploty"=w188:dbl[], "Namerene odpory"=w187:dbl[])
        n54 = Index Array(array=w193) -> (element=w191:dbl)  [unwired: 1 in]
        n55 = Index Array(array=w192) -> (element=w190:dbl)  [unwired: 1 in]
        n56 = call "temperature_calc.vi"("Sensor parameters"=w189, "proud"=w190, "napeti"=w191) -> ("Odpor"=w186:dbl, "teplota"=w185:dbl)  [unwired: 7 in]
        n57 = Insert Into Array(array=w188, new element=w185) -> (w183:dbl[])  [unwired: 1 in]
        n58 = Insert Into Array(array=w187, new element=w186) -> (w182:dbl[])  [unwired: 1 in]
        n59 = Bundle By Name(cluster=w184, "Namerene teploty"=w183, "Namerene odpory"=w182) -> (w157:T6)
        n60 = Unbundle By Name(w157) -> ("Nejistoty teplot"=w142:dbl[], "Namerene teploty"=w152:dbl[], "Pocet mereni na prumer"=w141:u32)
        n61 = Unbundle By Name(w157) -> ("Casy mereni"=w164:timestamp[], "Pocet mereni na prumer"=w158:u32, "Casy prumerovani"=w147:timestamp[])
        n62 = Unbundle By Name(w157) -> ("Namerene odpory"=w175:dbl[], "Prumery odporu"=w174:dbl[], "Pocet mereni na prumer"=w173:u32)
        n63 = Unbundle By Name(w157) -> ("Namerene teploty"=w172:dbl[], "Prumery teplot"=w171:dbl[], "Pocet mereni na prumer"=w170:u32)
        n64 = Unbundle By Name(w157) -> ("Namerene napeti"=w181:dbl[], "Prumery napeti"=w180:dbl[], "Pocet mereni na prumer"=w179:u32)
        n65 = Unbundle By Name(w157) -> ("Namerene proudy"=w178:dbl[], "Prumery proudu"=w177:dbl[], "Pocet mereni na prumer"=w176:u32)
        n66 = Array Size(array=w164) -> (size(s)=w139:i32)
        n67 = Array Size(array=w152) -> (size(s)=w137:i32)
        n68 = call "calc_running_avg.vi"("Size of batch"=w173, "Averages in"=w174, "Measure data"=w175) -> ("Averages out"=w167:dbl[])  [unwired: 8 in]
        n69 = call "calc_running_avg.vi"("Size of batch"=w179, "Averages in"=w180, "Measure data"=w181) -> ("Averages out"=w169:dbl[])  [unwired: 8 in]
        n70 = call "calc_running_avg.vi"("Size of batch"=w176, "Averages in"=w177, "Measure data"=w178) -> ("Averages out"=w168:dbl[])  [unwired: 8 in]
        n71 = call "calc_running_avg.vi"("Size of batch"=w170, "Averages in"=w171, "Measure data"=w172) -> ("Averages out"=w166:dbl[])  [unwired: 8 in]
        n72 = Decrement(x=w139) -> (x-1=w138:i32)
        n73 = Decrement(x=w137) -> (x-1=w136:i32)
        n74 = Quotient & Remainder(x=w138, y=w158) -> (floor(x/y)=w143:u32)  [unwired: 1 out]
        n75 = Quotient & Remainder(x=w136, y=w141) -> (floor(x/y)=w140:u32)  [unwired: 1 out]
        n76 = Multiply(x=w158, y=w143) -> (x*y=w144:u32)
        n77 = Multiply(x=w140, y=w141) -> (x*y=w149:u32)
        n78 = Index Array(array=w164, index=w144) -> (element=w159:timestamp)
        n79 = Index Array(array=w164, index=w138) -> (element=w163:timestamp)
        n80 = Array Subset(array=w152, index=w149) -> (w156:dbl[])  [unwired: 1 in]
        n81 = Subtract(x=w163, y=w159) -> (x-y=w162:dbl)
        n82 = call "type_A_uncertainty.vi"("X"=w156) -> ("u_A(x)"=w153:dbl)  [unwired: 9 in, 1 out]
        n83 = Divide(x=w162, y=2.0) -> (x/y=w160:dbl)
        n84 = Delete From Array(array=w142, length=1, index=w140) -> (array with subset deleted=w155:dbl[])  [unwired: 1 out]
        n85 = Add(x=w160, y=w159) -> (x+y=w146:timestamp)
        n86 = Insert Into Array(array=w155, new element=w153) -> (w151:dbl[])  [unwired: 1 in]
        n87 = Delete From Array(array=w147, length=1, index=w143) -> (array with subset deleted=w148:timestamp[])  [unwired: 1 out]
        n88 = Insert Into Array(array=w148, new element=w146) -> (w145:timestamp[])  [unwired: 1 in]
        n89 = Bundle By Name(cluster=w157, "Prumery napeti"=w169, "Prumery proudu"=w168, "Prumery odporu"=w167, "Prumery teplot"=w166, "Nejistoty teplot"=w151, "Casy prumerovani"=w145) -> (w165:T6)
      }
      frame "Display" {
        w201 = 0 ("index")
        w206 = State."Meas_done?"  # Initial State
        # "Bar"
        # "Graf"
        # "Tabulka"
        n90 = Unbundle By Name(w200) -> ("Casy mereni"=w197:timestamp[], "Celkovy pocet mereni"=w196:u32)
        n91 = Unbundle By Name(w200) -> ("Casy prumerovani"=w230:timestamp[], "Prumery napeti"=w234:dbl[], "Prumery proudu"=w221:dbl[], "Prumery odporu"=w220:dbl[], "Prumery teplot"=w219:dbl[], "Nejistoty teplot"=w202:dbl[])
        n92 = Unbundle By Name(w200) -> ("Casy prumerovani"=w214:timestamp[], "Prumery teplot"=w208:dbl[])
        n93 = for {
          tunnel: w230 -> [w238] mode=indexing
          tunnel: [w237] -> w229 mode=indexing
          n94 = Format Date/Time String(time format string (%c)="%c", seconds (now)=w238, UTC format=FALSE) -> (date/time string=w237:string)
        }
        n95 = Array Size(array=w197) -> (size(s)=w199:i32)
        n96 = Index Array(array=w214, index #1=1 ("index"), index #2=0 ("index")) -> (element #1=w211:timestamp, element #2=w209:timestamp)
        n97 = Divide(x=w199, y=w196) -> (x/y=→"Probiha mereni":dbl)
        n98 = Number To Fractional String(number=w234) -> (F-format string=w233:string[])  [unwired: 3 in]
        n99 = Number To Fractional String(number=w221) -> (F-format string=w227:string[])  [unwired: 3 in]
        n100 = Number To Fractional String(number=w220) -> (F-format string=w225:string[])  [unwired: 3 in]
        n101 = Number To Fractional String(number=w219) -> (F-format string=w223:string[])  [unwired: 3 in]
        n102 = Number To Fractional String(number=w202) -> (F-format string=w205:string[])  [unwired: 3 in]
        n103 = Subtract(x=w211, y=w209) -> (x-y=w210:dbl)
        n104 = Bundle By Name("dt"=w210, "t0"=w209, "Y"=w208) -> (→"Prumerna teplota":waveform(dbl))  [unwired: 1 in]
        n105 = Insert Into Array(array=w229, index=w201, new element="Casy prumeru" ("new element/subarray")) -> (w215:string[])
        n106 = Insert Into Array(array=w233, index=w201, new element="Prumery napeti [V]" ("new element/subarray")) -> (w231:string[])
        n107 = Insert Into Array(array=w227, index=w201, new element="Prumery proudu [A]" ("new element/subarray")) -> (w218:string[])
        n108 = Insert Into Array(array=w225, index=w201, new element="Prumery odporu [Ohm]" ("new element/subarray")) -> (w217:string[])
        n109 = Insert Into Array(array=w223, index=w201, new element="Prumery teploty [°C]" ("new element/subarray")) -> (w216:string[])
        n110 = Insert Into Array(array=w205, index=w201, new element="Nejistoty teplot [°C]" ("new element/subarray")) -> (w203:string[])
        n111 = Build Array(w215, w231, w218, w217, w216, w203) -> (→"Table":string[][])
      }
      frame "Meas_done?" {
        n112 = Unbundle By Name(w250) -> ("Namerene napeti"=w249:dbl[], "Celkovy pocet mereni"=w248:u32)
        n113 = Array Size(array=w249) -> (size(s)=w247:i32)
        n114 = Greater Or Equal?(x=w247, y=w248) -> (x >= y?=w242:bool)
        n115 = Or(x="Stop mereni", y=w242) -> (x .or. y?=w243:bool)
        n116 = Select(t=State."Meas_end", s=w243, f=State."Measure") -> (s? t:f=w246:T7)
      }
      frame "Meas_end" {
        w261 = FALSE ("Visible")
        w268 = State."High_level_math"  # Initial State
        # "Uvolneni komunikace"
        n117 = property on="Stop mereni" class="Bool"(error in=w258, "DisabledEnum"=T8."Disabled and Grayed Out" ("Disabled")) -> (error out=w259:errorcluster)  [unwired: 1 in, 1 out]
        n118 = property on="Start mereni" class="AbsTime (strict)"(error in=w259, "Visible"=w261) -> (error out=w262:errorcluster)  [unwired: 1 in, 1 out]
        n119 = property on="Odhad konce mereni" class="AbsTime (strict)"(error in=w262, "Visible"=w261) -> (error out=w263:errorcluster)  [unwired: 1 in, 1 out]
        n120 = Unbundle By Name(w265) -> ("VISA OUT 34450"=w267:refnum<visa-resource-name>, "VISA OUT 34401A"=w266:refnum<visa-resource-name>)
        n121 = property on="Probiha mereni" class="Slide (strict)"(error in=w263, "Visible"=w261) -> (error out=w254:errorcluster)  [unwired: 1 in, 1 out]
        n122 = VISA Close(VISA resource name=w267) -> (error out=w256:errorcluster)  [unwired: 1 in]
        n123 = VISA Close(VISA resource name=w266) -> (error out=w257:errorcluster)  [unwired: 1 in]
        n124 = property on="Start mereni" class="Bool"(error in=w254, "DisabledEnum"=T8."Enabled" ("Disabled")) -> (error out=w253:errorcluster)  [unwired: 1 in, 1 out]
        n125 = Merge Errors(w256, w257) -> (w255:errorcluster)
        n126 = Merge Errors(w255, w253) -> (w264:errorcluster)
      }
      frame "High_level_math" {
        w270 = State."Save_measure"  # Initial State
        # "REZERVNI STAV\nTento stav nebyl v projektu nikdy využit, ale sloužil by ke komplexnějším výpočtům, po tom co by jsme nasbíraly všechny naměřena data."
      }
      frame "Save_param" {
        w297 = State."Initialization"  # Initial State
        # "Uprava poctu mereni podle poctu mereni na prumer"
        # "AUTOMATICKE NASTAVENI MERICICH PRISTROJU"
        # "Pokud je pocet mereni za sekundu realny, nechavame ho byt.\nPokud je nerealny, zmenime na maximalni rychlost mereni."
        n127 = Unbundle By Name(w289) -> ("AUTOMATICKE NASTAVENI \nPARAMETRU"=w295:enum16{"OFF", "Presnost", "Rychlost"})
        n128 = Unbundle By Name(w289) -> ("Pocet mereni za sekundu"=w274:dbl, "Rozliseni 34450"=w311:enum16{"4_1/2 fast", "4_1/2 slow", "5_1/2 fast"}, "Rozliseni 34401A"=w310:T3)
        n129 = Unbundle By Name(w289) -> ("Celkovy pocet mereni"=w294:u32, "Pocet mereni na prumer"=w293:u32)
        n130 = Equal?(x=w295, y=T9."OFF") -> (x = y?=w308:bool)
        n131 = Select(t=T8."Enabled" ("Disabled"), s=w308, f=T8."Disabled and Grayed Out" ("Disabled")) -> (s? t:f=w285:T8)
        n132 = property on="Rozliseni 34401A" class="Enum (strict)"("DisabledEnum"=w285) -> (error out=w287:errorcluster)  [unwired: 2 in, 1 out]
        n133 = property on="Rozsah 34401A" class="Enum (strict)"("DisabledEnum"=w285) -> (error out=w286:errorcluster)  [unwired: 2 in, 1 out]
        n134 = Quotient & Remainder(x=w294, y=w293) -> (x-y*floor(x/y)=w292:u32)  [unwired: 1 out]
        n135 = call "Time_for_measure.vi"("Rozliseni 34401A"=w310, "Rozliseni 34450"=w311) -> ("Time for measure"=w302:u32)  [unwired: 9 in]
        n136 = Divide(x=w302, y=u32 1000) -> (x/y=w300:dbl)
        n137 = property on="Rozliseni 34450A" class="Enum (strict)"(error in=w287, "DisabledEnum"=w285) -> (error out=w284:errorcluster)  [unwired: 1 in, 1 out]
        n138 = property on="Rozsah 34450A" class="Enum (strict)"(error in=w286, "DisabledEnum"=w285) -> (error out=w283:errorcluster)  [unwired: 1 in, 1 out]
        n139 = Multiply(x=w292, y=w293) -> (x*y=w290:u32)
        n140 = Reciprocal(x=w300) -> (1/x=w273:dbl)
        n141 = Bundle By Name(cluster=w289, "Celkovy pocet mereni"=w290) -> (w288:T6)
        n142 = Less Or Equal?(x=w274, y=w273) -> (x <= y?=w276:bool)
        n143 = Merge Errors(w284, w283, w291) -> (w305:errorcluster)
        n144 = case shown="\"Presnost\"" w295 {
          tunnel: [w320 enum16{"4_1/2 fast", "4_1/2 slow", "5_1/2 fast"}."5_1/2 fast" ("Rozliseni 34450") enum16{"4_1/2 fast", "4_1/2 slow", "5_1/2 fast"}."4_1/2 fast" ("Rozliseni 34450")] -> w281
          tunnel: [w321 T2."10 V" ("Value") T2."10 V" ("Value")] -> w280
          tunnel: [w322 T3."6_1/2 slow" ("Value") T3."4_1/2 fast" ("Value")] -> w279
          tunnel: [w316 errorcluster {"status"=FALSE, "code"=0, "source"=""} ("error constant") errorcluster {"status"=FALSE, "code"=0, "source"=""} ("error constant")] -> w304
          tunnel: [w323 enum16{"10 mA", "100 mA", "1 A", "3 A"}."10 mA" ("Rozsah 34401A 2") enum16{"10 mA", "100 mA", "1 A", "3 A"}."10 mA" ("Rozsah 34401A 2")] -> w277
          frame "OFF", Default {
            n145 = property on="Rozliseni 34450A" class="Enum (strict)"() -> (error out=w319:errorcluster, "Value"=w320:enum16{"4_1/2 fast", "4_1/2 slow", "5_1/2 fast"})  [unwired: 2 in, 1 out]
            n146 = property on="Rozsah 34450A" class="Enum (strict)"(error in=w319) -> (error out=w318:errorcluster, "Value"=w321:T2)  [unwired: 1 in, 1 out]
            n147 = property on="Rozliseni 34401A" class="Enum (strict)"(error in=w318) -> (error out=w317:errorcluster, "Value"=w322:T3)  [unwired: 1 in, 1 out]
            n148 = property on="Rozsah 34401A" class="Enum (strict)"(error in=w317) -> (error out=w316:errorcluster, "Value"=w323:enum16{"10 mA", "100 mA", "1 A", "3 A"})  [unwired: 1 in, 1 out]
          }
          frame "Presnost" {
          }
          frame "Rychlost" {
          }
        }
        n149 = case shown="True" w276 {
          tunnel: [w313 w315] -> w275
          tunnel: w274 -> [_ w315]
          tunnel: w273 -> [w313 _]
          tunnel: [w312 errorcluster {"status"=FALSE, "code"=0, "source"=""} ("error constant")] -> w272
          frame False {
            n150 = property on="Pocet mereni za sekundu" class="DigNum (strict)"("Value"=w313) -> (error out=w312:errorcluster)  [unwired: 2 in, 1 out]
          }
          frame True {
          }
        }
        n151 = Bundle By Name(cluster=w288, "Pocet mereni za sekundu"=w275) -> (w282:T6)
        n152 = Merge Errors(w272, w304, w305) -> (w303:errorcluster)
        n153 = Bundle By Name(cluster=w282, "Rozliseni 34450"=w281, "Rozsah 34450"=w280, "Rozliseni 34401A"=w279, "Rozsah 34401A"=w277) -> (w278:T6)
        n154 = Select(t=w297, s="Start mereni", f=State."Set_params") -> (s? t:f=w296:T7)
      }
      frame "Save_measure" {
        w336 = State."Set_params"  # Initial State
        n155 = case shown="0, Default" "Ukladani" {
          tunnel: w340 -> [w349 w478]
          tunnel: [w343 w419] -> w337
          tunnel: "Save measurement to:" -> [w350 w418]
          frame 0, Default {
            w345 = FALSE ("use system decimal point (T)")
            w364 = 0 ("index")
            w380 = FALSE ("use system decimal point (T)")
            w394 = 0 ("index")
            n156 = Unbundle By Name(w349) -> ("Casy mereni"=w409:timestamp[], "Namerene napeti"=w408:dbl[], "Namerene proudy"=w407:dbl[], "Namerene odpory"=w406:dbl[], "Namerene teploty"=w405:dbl[])
            n157 = Unbundle By Name(w349) -> ("Casy prumerovani"=w379:timestamp[], "Prumery napeti"=w378:dbl[], "Prumery proudu"=w377:dbl[], "Prumery odporu"=w376:dbl[], "Prumery teplot"=w375:dbl[], "Nejistoty teplot"=w346:dbl[])
            n158 = for {
              tunnel: [w415] -> w403 mode=indexing
              tunnel: w409 -> [w414] mode=indexing
              n159 = Format Date/Time String(time format string (%c)="%c", seconds (now)=w414, UTC format=FALSE) -> (date/time string=w415:string)
            }
            n160 = for {
              tunnel: [w411] -> w373 mode=indexing
              tunnel: w379 -> [w410] mode=indexing
              n161 = Format Date/Time String(time format string (%c)="%c", seconds (now)=w410, UTC format=FALSE) -> (date/time string=w411:string)
            }
            n162 = Number To Fractional String(use system decimal point (T)=w380, number=w408) -> (F-format string=w401:string[])  [unwired: 2 in]
            n163 = Number To Fractional String(use system decimal point (T)=w380, number=w407) -> (F-format string=w397:string[])  [unwired: 2 in]
            n164 = Number To Fractional String(use system decimal point (T)=w380, number=w406) -> (F-format string=w396:string[])  [unwired: 2 in]
            n165 = Number To Fractional String(use system decimal point (T)=w380, number=w405) -> (F-format string=w395:string[])  [unwired: 2 in]
            n166 = Number To Fractional String(use system decimal point (T)=w345, number=w378) -> (F-format string=w371:string[])  [unwired: 2 in]
            n167 = Number To Fractional String(use system decimal point (T)=w345, number=w377) -> (F-format string=w367:string[])  [unwired: 2 in]
            n168 = Number To Fractional String(use system decimal point (T)=w345, number=w376) -> (F-format string=w366:string[])  [unwired: 2 in]
            n169 = Number To Fractional String(use system decimal point (T)=w345, number=w375) -> (F-format string=w365:string[])  [unwired: 2 in]
            n170 = Number To Fractional String(use system decimal point (T)=w345, number=w346) -> (F-format string=w347:string[])  [unwired: 2 in]
            n171 = Insert Into Array(array=w401, index=w394, new element="Namerene napeti [V]" ("new element/subarray")) -> (w392:string[])
            n172 = Insert Into Array(array=w403, index=w394, new element="Casy mereni" ("new element/subarray")) -> (w393:string[])
            n173 = Insert Into Array(array=w397, index=w394, new element="Namerene proudy [A]" ("new element/subarray")) -> (w389:string[])
            n174 = Insert Into Array(array=w396, index=w394, new element="Namerene odpory [Ohm]" ("new element/subarray")) -> (w390:string[])
            n175 = Insert Into Array(array=w395, index=w394, new element="Namerene teploty [°C]" ("new element/subarray")) -> (w391:string[])
            n176 = Insert Into Array(array=w371, index=w364, new element="Prumery napeti [V]" ("new element/subarray")) -> (w362:string[])
            n177 = Insert Into Array(array=w373, index=w364, new element="Casy prumerovani" ("new element/subarray")) -> (w363:string[])
            n178 = Insert Into Array(array=w367, index=w364, new element="Prumery proudu [A]" ("new element/subarray")) -> (w359:string[])
            n179 = Insert Into Array(array=w366, index=w364, new element="Prumery odporu [Ohm]" ("new element/subarray")) -> (w360:string[])
            n180 = Insert Into Array(array=w365, index=w364, new element="Prumery teplot [°C]" ("new element/subarray")) -> (w361:string[])
            n181 = Insert Into Array(array=w347, new element="Nejistoty teplot [°C]" ("new element/subarray")) -> (w344:string[])  [unwired: 1 in]
            n182 = Build Array(w393, w392, w389, w390, w391) -> (w387:string[][])
            n183 = Build Array(w363, w362, w359, w360, w361, w344) -> (w357:string[][])
            n184 = Path To String(path=w350) -> (string=w383:string)
            n185 = Path To String(path=w350) -> (string=w353:string)
            n186 = Concatenate Strings(w383, "-hodnoty.csv" ("string")) -> (w382:string)
            n187 = call <vilib>:"Application Directory.vi"() -> ("Application Directory"=w388:path)
            n188 = Concatenate Strings(w353, "-prumery.csv" ("string")) -> (w352:string)
            n189 = call <vilib>:"Application Directory.vi"() -> ("Application Directory"=w358:path)
            n190 = Build Path(base path=w388, name or relative path=w382) -> (appended path=w384:path)
            n191 = Build Path(base path=w358, name or relative path=w352) -> (appended path=w354:path)
            n192 = call-poly <vilib>:"Write Delimited Spreadsheet.vi"("file path (dialog if empty)"=w384, "2D data"=w387, "transpose? (no:F)"=TRUE, "delimiter (\\t)"="," ("delimiter (\\t)")) -> ("error out"=w342:errorcluster)  [unwired: 10 in, 1 out]
            n193 = call-poly <vilib>:"Write Delimited Spreadsheet.vi"("file path (dialog if empty)"=w354, "2D data"=w357, "transpose? (no:F)"=TRUE, "delimiter (\\t)"="," ("delimiter (\\t)")) -> ("error out"=w341:errorcluster)  [unwired: 10 in, 1 out]
            n194 = Merge Errors(w342, w341) -> (w343:errorcluster)
          }
          frame 1 {
            n195 = call <vilib>:"Application Directory.vi"() -> ("Application Directory"=w480:path)
            n196 = Unbundle By Name(w478) -> ("Namerene napeti"=w477:dbl[], "Namerene proudy"=w472:dbl[], "Namerene odpory"=w467:dbl[], "Namerene teploty"=w463:dbl[], "Prumery napeti"=w450:dbl[], "Prumery proudu"=w449:dbl[], "Prumery odporu"=w448:dbl[], "Prumery teplot"=w447:dbl[], "Casy mereni"=w434:timestamp[], "Casy prumerovani"=w433:timestamp[], "Nejistoty teplot"=w427:dbl[])
            n197 = Build Path(base path=w480, name or relative path=w418) -> (appended path=w425:path)
            n198 = Path To String(path=w418) -> (string=w479:string)
            n199 = TDMS Open(10:T10."create or replace" ("operation (0:open)"), 11:w425) -> (0:w423:errorcluster, 3:w424:refnum<k34>)  [unwired: 5 in]
            n200 = TDMS Write(0:w424, 5:w479, 7:string[] ["Voltage [V]"] ("channel name(s) in (Untitled)"), 9:w477, 11:w423) -> (4:w475:refnum<k34>, 6:w474:string, 15:w473:errorcluster)  [unwired: 1 in, 1 out]
            n201 = TDMS Write(0:w475, 5:w474, 7:string[] ["Current [A]"] ("channel name(s) in (Untitled)"), 9:w472, 11:w473) -> (4:w470:refnum<k34>, 6:w469:string, 15:w468:errorcluster)  [unwired: 1 in, 1 out]
            n202 = TDMS Write(0:w470, 5:w469, 7:string[] ["Resistance [Ohm]"] ("channel name(s) in (Untitled)"), 9:w467, 11:w468) -> (4:w466:refnum<k34>, 6:w465:string, 15:w464:errorcluster)  [unwired: 1 in, 1 out]
            n203 = TDMS Write(0:w466, 5:w465, 7:string[] ["Temperature [°C]"] ("channel name(s) in (Untitled)"), 9:w463, 11:w464) -> (4:w462:refnum<k34>, 6:w461:string, 15:w460:errorcluster)  [unwired: 1 in, 1 out]
            n204 = TDMS Write(0:w462, 5:w461, 7:string[] ["Voltage averages [V]"] ("channel name(s) in (Untitled)"), 9:w450, 11:w460) -> (4:w459:refnum<k34>, 6:w458:string, 15:w457:errorcluster)  [unwired: 1 in, 1 out]
            n205 = TDMS Write(0:w459, 5:w458, 7:string[] ["Current averages [A]"] ("channel name(s) in (Untitled)"), 9:w449, 11:w457) -> (4:w456:refnum<k34>, 6:w455:string, 15:w454:errorcluster)  [unwired: 1 in, 1 out]
            n206 = TDMS Write(0:w456, 5:w455, 7:string[] ["Resistance averages [Ohm]"] ("channel name(s) in (Untitled)"), 9:w448, 11:w454) -> (4:w453:refnum<k34>, 6:w452:string, 15:w451:errorcluster)  [unwired: 1 in, 1 out]
            n207 = TDMS Write(0:w453, 5:w452, 7:string[] ["Temperature averages [°C]"] ("channel name(s) in (Untitled)"), 9:w447, 11:w451) -> (4:w440:refnum<k34>, 6:w439:string, 15:w438:errorcluster)  [unwired: 1 in, 1 out]
            n208 = TDMS Write(0:w440, 5:w439, 7:string[] ["Measurement times"] ("channel name(s) in (Untitled)"), 9:w434, 11:w438) -> (4:w437:refnum<k34>, 6:w436:string, 15:w435:errorcluster)  [unwired: 1 in, 1 out]
            n209 = TDMS Write(0:w437, 5:w436, 7:string[] ["Times of averaging"] ("channel name(s) in (Untitled)"), 9:w433, 11:w435) -> (4:w430:refnum<k34>, 6:w429:string, 15:w428:errorcluster)  [unwired: 1 in, 1 out]
            n210 = TDMS Write(0:w430, 5:w429, 7:string[] ["Temperature uncertainty [°C]"] ("channel name(s) in (Untitled)"), 9:w427, 11:w428) -> (4:w420:refnum<k34>, 15:w421:errorcluster)  [unwired: 1 in, 2 out]
            n211 = TDMS Close(8:w421, 11:w420) -> (0:w419:errorcluster)  [unwired: 1 out]
          }
        }
        n212 = Merge Errors(w337, w339) -> (w338:errorcluster)
      }
      frame "Set_params" {
        n213 = Bundle By Name(cluster=w498, "Sensor parameters"="Sensor parameters", "VISA resource name 34401A"="VISA resource name 34401A", "Serial Settings 34401A"="Serial Settings 34401A", "Delay before read 34401A"="delay before read 34401A", "VISA resource name 34450"="VISA resource name 34450A", "Delay before read 34450"="delay before read 34450A", "Pocet mereni za sekundu"="Pocet mereni za sekundu", "Celkovy pocet mereni"="Celkovy pocet mereni", "Pocet mereni na prumer"="Pocet mereni na prumer", "Rozliseni 34450"="Rozliseni 34450A", "Rozsah 34450"="Rozsah 34450A", "Rozliseni 34401A"="Rozliseni 34401A", "Rozsah 34401A"="Rozsah 34401A", "AUTOMATICKE NASTAVENI \nPARAMETRU"="AUTOMATICKE NASTAVENI \nPARAMETRU") -> (w497:T6)
      }
    }
    n214 = Or(x=w15, y="stop") -> (x .or. y?=w19:bool)
  }
  n215 = Unbundle By Name(w7) -> ("VISA OUT 34450"=w6:refnum<visa-resource-name>, "VISA OUT 34401A"=w5:refnum<visa-resource-name>)
  n216 = VISA Close(VISA resource name=w6) -> (error out=w1:errorcluster)  [unwired: 1 in]
  n217 = VISA Close(VISA resource name=w5) -> (error out=w2:errorcluster)  [unwired: 1 in]
  n218 = Merge Errors(w1, w2, w4) -> (w3:errorcluster)
  n219 = call <vilib>:"Simple Error Handler.vi"("error in (no error)"=w3) -> ("error out"=w9:errorcluster)  [unwired: 4 in, 4 out]
  n220 = disable-structure shown="Default" {
    disable-tunnel: w9 -> [_ _]
    frame condition #0 (active) {
    }
    frame condition #1 {
      # "Call Quit LabVIEW if running as a built application."
      n221 = Quit LabVIEW() -> ()  [unwired: 1 in]
    }
  }
